vi "Query ID.vi"(8 "error in (no error)":errorcluster, 10 "Query String(*IDN?)":string="*IDN?", 11 "CS in":refnum<class "QCS.lvclass">) -> (0 "error out":errorcluster, 2 "ID  string":string, 3 "CS out":refnum<class "QCS.lvclass">)   [LabVIEW 2019, in "QCS.lvclass"]
uses:
  Lib.llb/QCS.lvclass
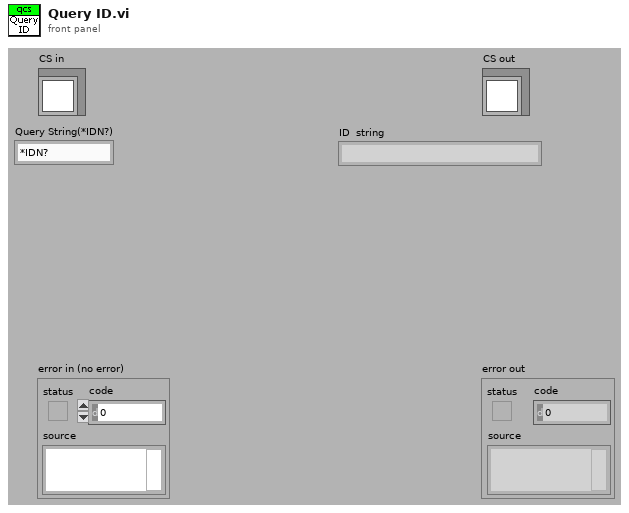
[diagram p1: front panel]
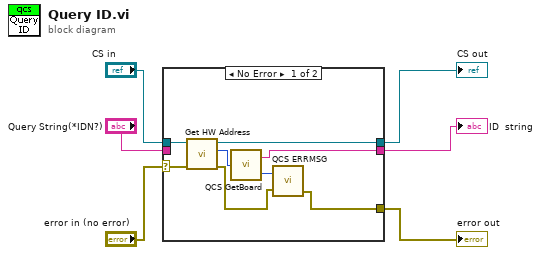
[diagram p0: block diagram]
diagram:
  n1 = case shown="No Error" "error in (no error)" {
    selector: "error in (no error)" -> [w11 w15]
    tunnel: [w7 w15] -> w6
    tunnel: [w14 _] -> w5
    tunnel: [w12 w16] -> w4
    tunnel: "Query String(*IDN?)" -> [_ _]
    tunnel: "CS in" -> [w13 w16]
    frame No Error {
      n2 = call-dynamic "Get HW Address.vi"("error in (no error)"=w11, "CS.lvclass in"=w13) -> ("error out"=w8:errorcluster, "HW Address"=w10:i32, "CS.lvclass out"=w12:refnum<class "QCS.lvclass">)  [unwired: 7 in]
      n3 = call "QCS GetBoard.VI"("BoardNum"=w10) -> ("Board Name"=w14:string, "ErrCode"=w9:i32)
      n4 = call "QCS ERRMSG.VI"("ErrCode"=w9, "error in (no error)"=w8) -> ("error out"=w7:errorcluster)  [unwired: 2 out]
    }
    frame Error {
    }
  }
  "error out" <- w6
  "CS out" <- w4
  "ID  string" <- w5
